vi "环形数据队列(CDB).vi"(8 "error in (no error)":errorcluster caption="错误输入（无错误）", 9 "重置":bool, 10 "队列长度":i32=8, 11 "输入数据":cdb) -> (0 "error out":errorcluster caption="错误输出", 1 "队列满":bool, 2 "出队元素":cdb, 3 "预览队列":cdb[](array[numeric]))   [LabVIEW 2011]
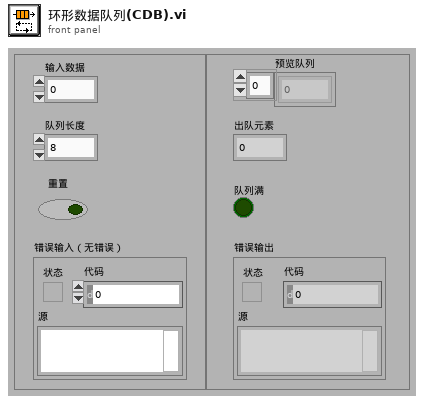
[diagram p1: front panel]
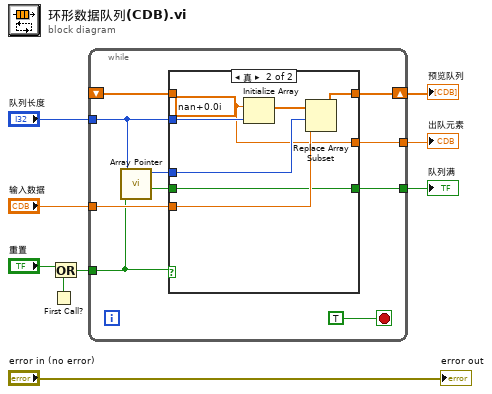
[diagram p0: block diagram]
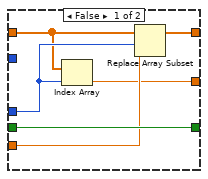
[diagram p2: hidden frame]
diagram:
  n1 = First Call?() -> (First Call?: T/F=w7:bool)
  n2 = Or(x="重置", y=w7) -> (x .or. y?=w6:bool)
  n3 = while {
    shift-right: [w18] -> w2
    shift-left: _ -> [w17]
    tunnel: "队列长度" -> [w15]
    tunnel: w6 -> [w14]
    tunnel: "输入数据" -> [w16]
    tunnel: [w11] -> w4
    tunnel: [w10] -> w3
    stop <- TRUE stop-if-true
    n4 = call "Array Pointer.vi"("Size"=w15, "Reset"=w14) -> ("Full"=w12:bool, "Current Pos"=w13:i32)  [unwired: 6 in, 2 out]
    n5 = case shown="真" w14 {
      tunnel: w15 -> [_ w32]
      tunnel: [w24 w30] -> w18
      tunnel: w17 -> [w21 _]
      tunnel: w16 -> [w23 w29]
      tunnel: w13 -> [w22 w28]
      tunnel: w12 -> [w25 w27]
      tunnel: [w25 w27] -> w11
      tunnel: [w20 w26] -> w10
      frame False {
        n6 = Index Array(array=w21, index=w22) -> (element=w20:cdb)
        n7 = Replace Array Subset(array=w21, new element=w23, index=w22) -> (w24:cdb[])
      }
      frame True {
        w26 = cdb nan+0.0i ("元素")
        n8 = Initialize Array(w26, w32) -> (w31:cdb[])
        n9 = Replace Array Subset(array=w31, new element=w29, index=w28) -> (w30:cdb[])
      }
    }
  }
  "队列满" <- w4
  "出队元素" <- w3
  "预览队列" <- w2
  "error out" <- "error in (no error)"
